vi "convertTableToArray.vi"(8 "error in":errorcluster, 11 "tbl":string[][](array[string])) -> (0 "error out":errorcluster, 3 "contArr":string[](array[string]))   [LabVIEW 2010]
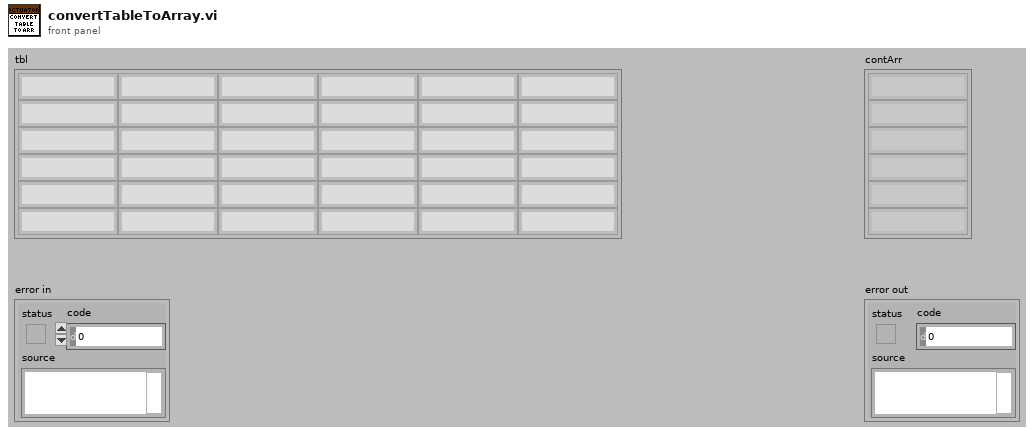
[diagram p1: front panel]
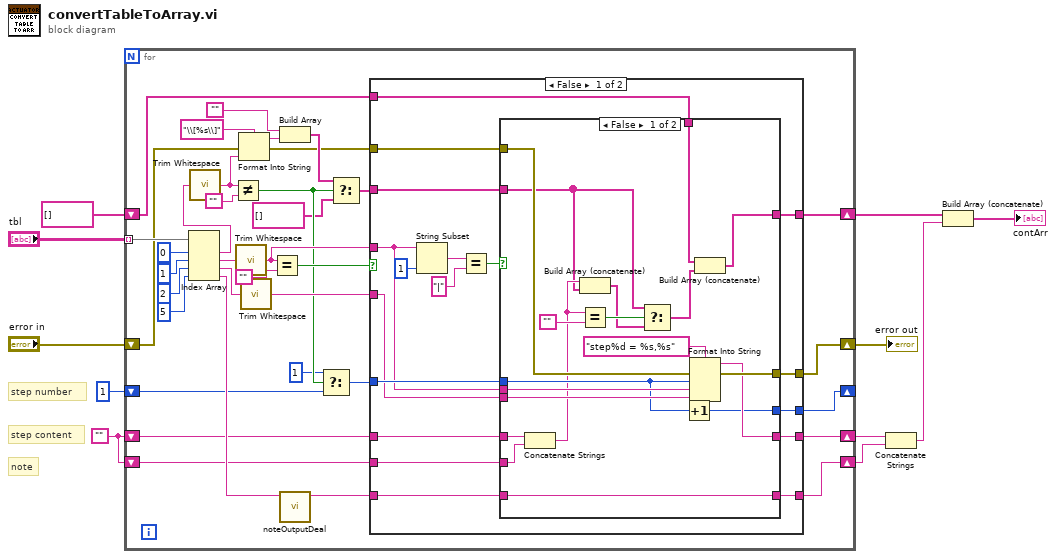
[diagram p0: block diagram]
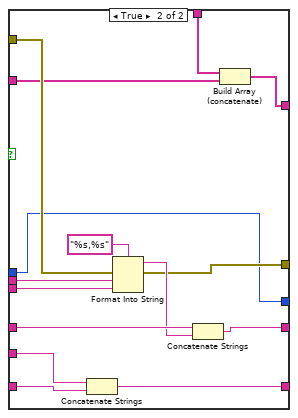
[diagram p2: hidden frame]
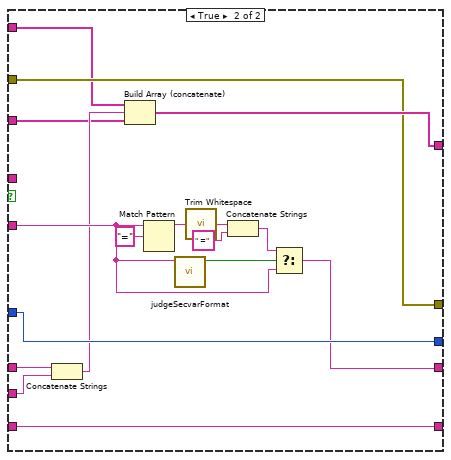
[diagram p3: hidden frame]
diagram:
  w6 = ""
  # "note"
  # "step content"
  # "step number"
  n1 = for {
    tunnel: "tbl" -> [w46] mode=indexing
    shift-right: [w21] -> w3
    shift-left: string[] [] ("Value") -> [w12]
    shift-right: [w19] -> w7
    shift-left: "error in" -> [w32]
    shift-right: [w14] -> _
    shift-left: 1 ("input 1") -> [w16]
    shift-right: [w26] -> w5
    shift-left: w6 -> [w24]
    shift-right: [w25] -> w4
    shift-left: w6 -> [w23]
    n2 = Index Array(array=w46, index #1=0 ("index"), index #2=1 ("index"), index #3=2 ("index"), index #4=5 ("index")) -> (element #1=w36:string, element #2=w42:string, element #3=w40:string, element #4=w39:string)
    n3 = call <vilib>:"Trim Whitespace.vi"("string"=w36) -> ("trimmed string"=w35:string)  [unwired: 1 in]
    n4 = Not Equal?(x=w35, y="") -> (x != y?=w18:bool)
    n5 = call <vilib>:"Trim Whitespace.vi"("string"=w42) -> ("trimmed string"=w28:string)  [unwired: 1 in]
    n6 = Format Into String(format string="\\[%s\\]", error in=w32, w35) -> (resulting string=w34:string, error out=w20:errorcluster)  [unwired: 1 in]
    n7 = call <vilib>:"Trim Whitespace.vi"("string"=w40) -> ("trimmed string"=w27:string)  [unwired: 1 in]
    n8 = Equal?(x=w28, y="") -> (x = y?=w31:bool)
    n9 = Build Array("", w34) -> (w33:string[])
    n10 = call "noteOutputDeal.vi"("note in editor"=w39) -> ("note output"=w29:string)  [unwired: 10 in]
    n11 = Select(t=1 ("input 1"), s=w18, f=w16) -> (s? t:f=w15:i32)
    n12 = Select(t=w33, s=w18, f=string[] [] ("Value")) -> (s? t:f=w22:string[])
    n13 = case shown="False" w31 {
      tunnel: w29 -> [w56 w104]
      tunnel: w15 -> [w61 w116]
      tunnel: w28 -> [w60 _]
      tunnel: w27 -> [w59 w106]
      tunnel: [w58 w105] -> w26
      tunnel: [w55 w104] -> w25
      tunnel: w24 -> [w57 w115]
      tunnel: w23 -> [w54 w114]
      tunnel: w22 -> [w53 w101]
      tunnel: [w52 w113] -> w21
      tunnel: w20 -> [w51 w103]
      tunnel: [w50 w103] -> w19
      tunnel: [w49 w116] -> w14
      tunnel: w12 -> [w48 w100]
      frame False {
        n14 = String Subset(string=w60, length (rest)=1 ("length (rest)")) -> (substring=w64:string)  [unwired: 1 in]
        n15 = Equal?(x=w64, y="|" ("format string")) -> (x = y?=w62:bool)
        n16 = case shown="False" w62 {
          tunnel: w61 -> [w75 w88]
          tunnel: w60 -> [w83 w98]
          tunnel: w59 -> [w82 w97]
          tunnel: [w76 w91] -> w58
          tunnel: w57 -> [w78 w93]
          tunnel: [w81 w94] -> w55
          tunnel: w56 -> [w81 w95]
          tunnel: w54 -> [w77 w96]
          tunnel: w53 -> [w69 w86]
          tunnel: [w66 w85] -> w52
          tunnel: w51 -> [w80 w90]
          tunnel: [w79 w89] -> w50
          tunnel: [w74 w88] -> w49
          tunnel: w48 -> [w67 w87]
          frame False {
            n17 = Concatenate Strings(w78, w77) -> (w70:string)
            n18 = Build Array (concatenate)(w70, w69) -> (w71:string[])
            n19 = Equal?(x=w70, y="") -> (x = y?=w72:bool)
            n20 = Select(t=w69, s=w72, f=w71) -> (s? t:f=w68:string[])
            n21 = Increment(x=w75) -> (x+1=w74:i32)
            n22 = Format Into String(format string="step%d = %s,%s", error in=w80, w75, w83, w82) -> (resulting string=w76:string, error out=w79:errorcluster)  [unwired: 1 in]
            n23 = Build Array (concatenate)(w67, w68) -> (w66:string[])
          }
          frame True {
            n24 = Concatenate Strings(w96, w95) -> (w94:string)
            n25 = Format Into String(format string="%s,%s", error in=w90, w98, w97) -> (resulting string=w92:string, error out=w89:errorcluster)  [unwired: 1 in]
            n26 = Concatenate Strings(w93, w92) -> (w91:string)
            n27 = Build Array (concatenate)(w87, w86) -> (w85:string[])
          }
        }
      }
      frame True {
        n28 = Concatenate Strings(w115, w114) -> (w102:string)
        n29 = Build Array (concatenate)(w100, w102, w101) -> (w113:string[])
        n30 = Match Pattern(string=w106, regular expression="=") -> (before substring=w109:string)  [unwired: 1 in, 3 out]
        n31 = call "judgeSecvarFormat.vi"("section variable"=w106) -> ("correct format?"=w107:bool)  [unwired: 10 in]
        n32 = call <vilib>:"Trim Whitespace.vi"("string"=w109) -> ("trimmed string"=w110:string)  [unwired: 1 in]
        n33 = Concatenate Strings(w110, " =" ("format string")) -> (w112:string)
        n34 = Select(t=w112, s=w107, f=w106) -> (s? t:f=w105:string)
      }
    }
  }
  "error out" <- w7
  n35 = Concatenate Strings(w5, w4) -> (w2:string)
  n36 = Build Array (concatenate)(w3, w2) -> (→"contArr":string[])
